vi "instantiate stream page.vi"(8 "error in (no error)":errorcluster, 11 "stream":T1 format="%.0x") -> (0 "error out":errorcluster)   [LabVIEW 2026, in "Nominal Core Streaming System Explorer.lvlib"]
uses:
  Nominal Core Streaming System Explorer.lvlib
  <vilib>/NI VeriStand/Custom Device API/Custom Device Item Ref.ctl
  <vilib>/NI VeriStand/Custom Device API/Custom Device Channel.ctl
  <vilib>/NI VeriStand/Custom Device API/Custom Device Channel Type.ctl
  Shared/Constants.vi
  Shared/Nominal Core Streaming Shared.lvlib
  <vilib>/NI VeriStand/Custom Device API/Custom Device API.lvlib
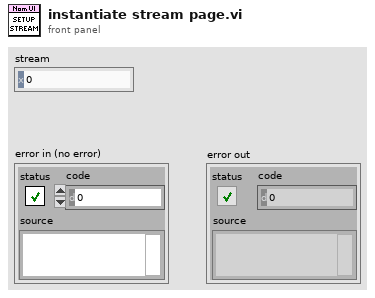
[diagram p1: front panel]
types:
  T1 = typedef "Custom Device API.lvlib/Custom Device Item Ref.ctl" = u64
  T2 = typedef "Custom Device API.lvlib/Custom Device Channel.ctl" = cluster{"Type":T3, "Units":string, "Default Value":dbl, "Faultable":bool, "Scalable":bool}
  T3 = typedef "Custom Device API.lvlib/Custom Device Channel Type.ctl" = enum16{"Input", "Output"}
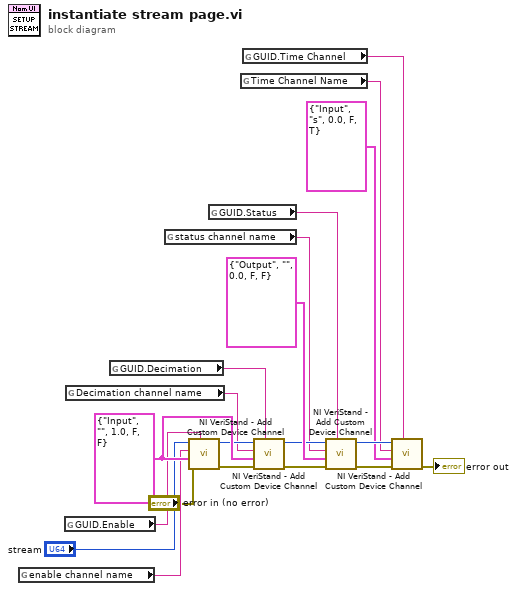
[diagram p0: block diagram]
diagram:
  w17 = T2 {"Type"=enum."Input", "Units"="", "Default Value"=1.0, "Faultable"=FALSE, "Scalable"=FALSE} ("Channel")
  n1 = global read "Constants.vi" "enable channel name"() -> (w11:string)
  n2 = global read "Constants.vi" "GUID.Enable"() -> (w1:string)
  n3 = global read "Constants.vi" "Decimation channel name"() -> (w10:string)
  n4 = global read "Constants.vi" "GUID.Decimation"() -> (w16:string)
  n5 = global read "Constants.vi" "status channel name"() -> (w9:string)
  n6 = call <vilib>:"NI VeriStand - Add Custom Device Channel.vi"("GUID (Default Channel)"=w1, "error in (no error)"="error in (no error)", "Channel"=w17, "Channel Name"=w11, "Parent Ref in"="stream") -> ("error out"=w18:errorcluster, "Parent Ref out"=w14:T1)  [unwired: 3 in, 2 out]
  n7 = global read "Constants.vi" "GUID.Status"() -> (w12:string)
  n8 = global read "Constants.vi" "Time Channel Name"() -> (w4:string)
  n9 = global read "Constants.vi" "GUID.Time Channel"() -> (w5:string)
  n10 = call <vilib>:"NI VeriStand - Add Custom Device Channel.vi"("GUID (Default Channel)"=w16, "error in (no error)"=w18, "Channel"=w17, "Channel Name"=w10, "Parent Ref in"=w14) -> ("error out"=w15:errorcluster, "Parent Ref out"=w19:T1)  [unwired: 3 in, 2 out]
  n11 = call <vilib>:"NI VeriStand - Add Custom Device Channel.vi"("GUID (Default Channel)"=w12, "error in (no error)"=w15, "Channel"=T2 {"Type"=enum."Output", "Units"="", "Default Value"=0.0, "Faultable"=FALSE, "Scalable"=FALSE}, "Channel Name"=w9, "Parent Ref in"=w19) -> ("error out"=w8:errorcluster, "Parent Ref out"=w6:T1)  [unwired: 3 in, 2 out]
  n12 = call <vilib>:"NI VeriStand - Add Custom Device Channel.vi"("GUID (Default Channel)"=w5, "error in (no error)"=w8, "Channel"=T2 {"Type"=enum."Input", "Units"="s", "Default Value"=0.0, "Faultable"=FALSE, "Scalable"=TRUE}, "Channel Name"=w4, "Parent Ref in"=w6) -> ("error out"=→"error out":errorcluster)  [unwired: 3 in, 3 out]
